vi "Init.vi"(8 "error in (no error)":errorcluster, 11 "Input Kind":string) -> (0 "error out":errorcluster, 3 "GetInputDefaultSettings out":refnum<class "GetInputDefaultSettings.lvclass">)   [LabVIEW 2022 SP3, in "obs-websocket-lv.lvlib" / "GetInputDefaultSettings.lvclass"]
uses:
  GetInputDefaultSettings.lvclass
  GetInputDefaultSettings.lvclass/GetInputDefaultSettings.ctl
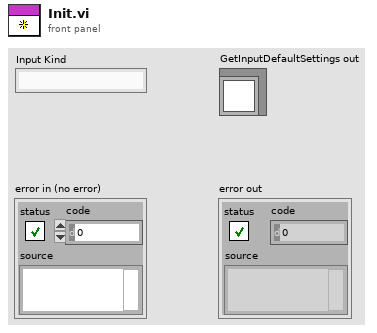
[diagram p1: front panel]
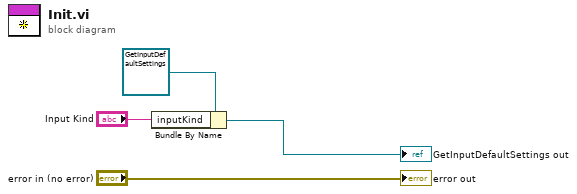
[diagram p0: block diagram]
diagram:
  n1 = Bundle By Name(cluster=refnum<class "GetInputDefaultSettings.lvclass"> refnum ("GetInputDefaultSettings in"), "inputKind"="Input Kind") -> (→"GetInputDefaultSettings out":refnum<class "GetInputDefaultSettings.lvclass">)
  "error out" <- "error in (no error)"
